vi "mapping to tag and channel name.vi"(10 "channel classification":T2, 11 "mapping":T1) -> (2 "tag":string, 3 "channel":string)   [LabVIEW 2013, in "engine configuration.lvclass"]
uses:
  engine configuration.lvclass
  <vilib>/NI/Tag Bus Module Framework/channel/channel classification.ctl
  <vilib>/NI/Tag Bus/table/mapping.ctl
  <vilib>/NI/Tag Bus Module Framework/channel/TBM channel.lvclass
  <vilib>/NI/Tag Bus/table/data table.lvlib
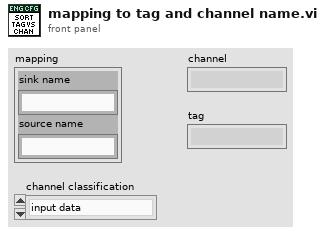
[diagram p1: front panel]
types:
  T1 = typedef "tag bus.lvlib/data table.lvlib/mapping.ctl" = cluster{"sink name":string, "source name":string}
  T2 = typedef "TBM channel.lvclass/channel classification.ctl" = enum16{"input data", "output data", "processing parameter", "processing result"}
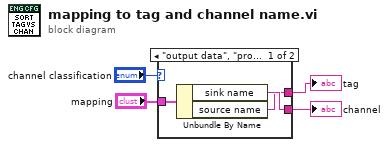
[diagram p0: block diagram]
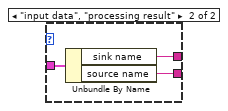
[diagram p2: hidden frame]
diagram:
  n1 = case shown="\"output data\", \"processing parameter\"" "channel classification" {
    tunnel: "mapping" -> [w7 w10]
    tunnel: [w6 w9] -> w3
    tunnel: [w5 w8] -> w4
    frame "output data", "processing parameter" {
      n2 = Unbundle By Name(w7) -> ("sink name"=w6:string, "source name"=w5:string)
    }
    frame "input data", "processing result" {
      n3 = Unbundle By Name(w10) -> ("sink name"=w8:string, "source name"=w9:string)
    }
  }
  "tag" <- w4
  "channel" <- w3
